vi "EvaluateLowRate.vi"(7 "Qbus":refnum<class "Qbus.lvclass">, 8 "error in (no error)":errorcluster, 9 "data":T1, 10 "new block number":u32, 11 "config":variant) -> (0 "error out":errorcluster, 1 "new data":T1, 2 "fire low rate data flow":bool, 3 "config out":variant)   [LabVIEW 2017, in "DataAccumulator.lvlib"]
uses:
  <vilib>/addons/InsightCM/Devices/Shared/Common/DataAccumulator/DataAccumulator.lvlib
  <vilib>/addons/InsightCM/Devices/Shared/Common/DataFlow/controls/Data.ctl
  <vilib>/addons/InsightCM/Utilities/DataAccessors/controls/wfmSGL_DVR.ctl
  <vilib>/addons/PointValueMap/controls/PointMap.ctl
  <vilib>/addons/InsightCM/Devices/Shared/Common/DataFlow/controls/Type.ctl
  <vilib>/addons/Qbus/Qbus.lvclass
  <vilib>/addons/InsightCM/Devices/Shared/Common/DataAccumulator/controls/DataStoreOps.ctl
  <vilib>/addons/InsightCM/Devices/Shared/Common/DVRBuffer/controls/BufferLocation.ctl
  <vilib>/addons/InsightCM/Devices/Shared/Common/DataAccumulator/controls/DataStoreType.ctl
  <vilib>/addons/InsightCM/Utilities/Analysis/Shared/controls/PulsePositions.ctl
  <vilib>/addons/InsightCM/Devices/Shared/Common/DataAccumulator/controls/BlockParams.ctl
  <vilib>/addons/InsightCM/Devices/Shared/Common/DVRBuffer/DVRBuffer.lvlib
  <vilib>/addons/PointValueMap/PointValueMap.lvlib
  <vilib>/addons/InsightCM/Devices/Shared/Common/DataFlow/DataFlow.lvlib
  <vilib>/addons/InsightCM/Utilities/Analysis/Shared/AnalysisHelper.lvlib
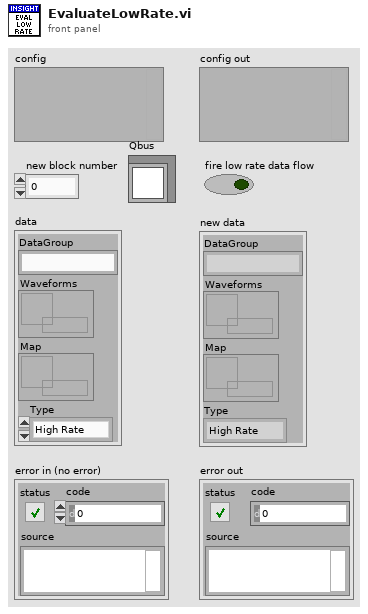
[diagram p1: front panel]
types:
  T1 = typedef "DataFlow.lvlib/Data.ctl" = cluster{"DataGroup":string, "Waveforms":T2, "Map":T3, "Type":T4}
  T2 = typedef "wfmSGL_DVR.ctl" = refnum<data-value>
  T3 = typedef "PointValueMap.lvlib/PointMap.ctl" = refnum<data-value>
  T4 = typedef "DataFlow.lvlib/Type.ctl" = enum16{"High Rate", "Low Rate", "Burst Mode"}
  T5 = typedef "DataAccumulator.lvlib/AccumulationSettings.ctl" = cluster{"Type":T6, "Length":dbl, "Max Time (sec)":dbl, "Start Block":T7, "Acquired (sec)":dbl, "Acquired (pulses)":i32, "Initial Pulse Offset":dbl, "Stop Block":T7, "LastBlockAdded":u32}
  T6 = typedef "DataAccumulator.lvlib/accumulationType.ctl" = enum16{"none", "seconds", "revolutions"}
  T7 = typedef "DVRBuffer.lvlib/BufferLocation.ctl" = cluster{"Block":u32, "Index":i32}
  T8 = typedef "DataAccumulator.lvlib/DataStoreOps.ctl" = enum16{"Reset", "Init", "Clear", "SetWfms", "GetWfms"}
  T9 = typedef "DataAccumulator.lvlib/DataStoreType.ctl" = cluster{"Group":string, "waveforms":waveform(sgl)[], "pulse positions array":T10[], "start block":T7}
  T10 = typedef "AnalysisHelper.lvlib/PulsePositions.ctl" = cluster{"Name":string, "Pulse Position Data":dbl[], "Pulses Per Rev":i32}
  T11 = typedef "DataAccumulator.lvlib/BlockParams.ctl" = cluster{"start block":T7, "stop block":T7, "BlockSizeSeconds":dbl}
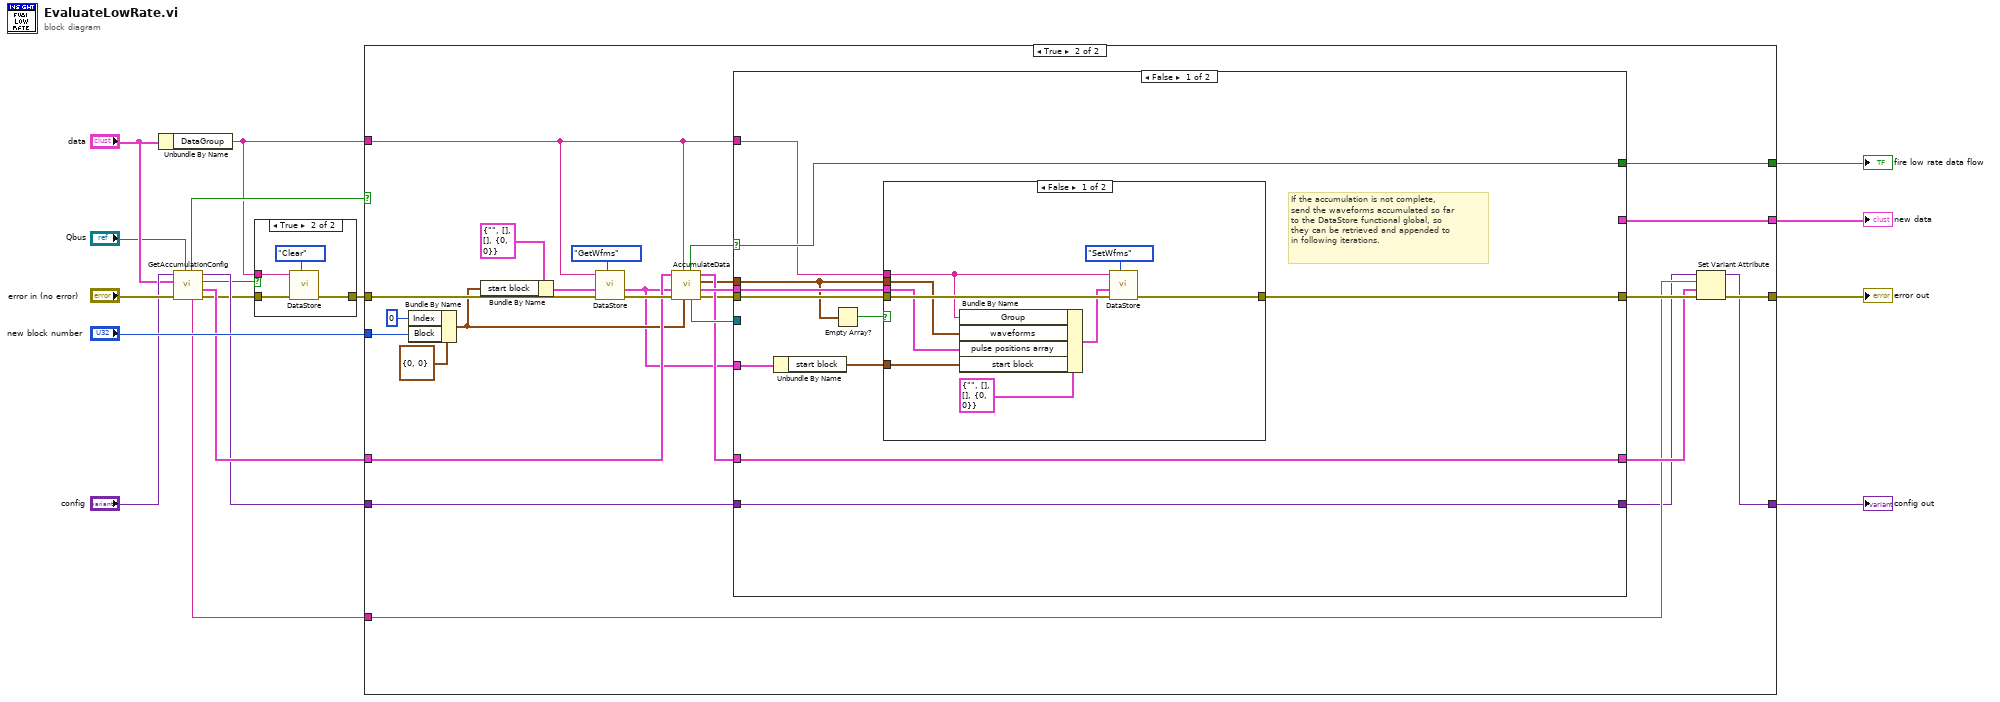
[diagram p0: block diagram]
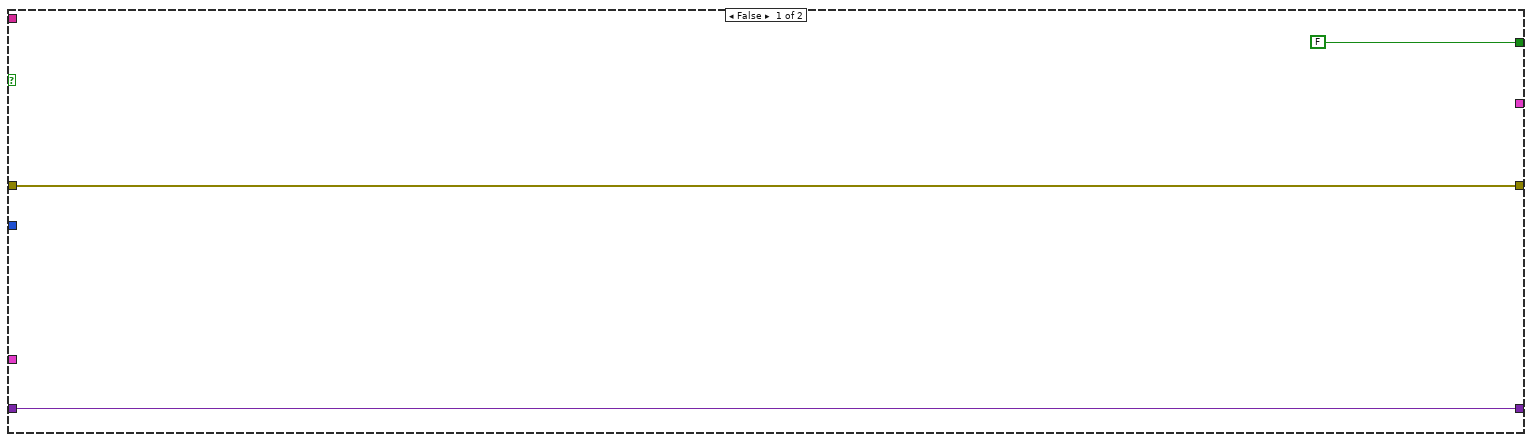
[diagram p2: hidden frame]
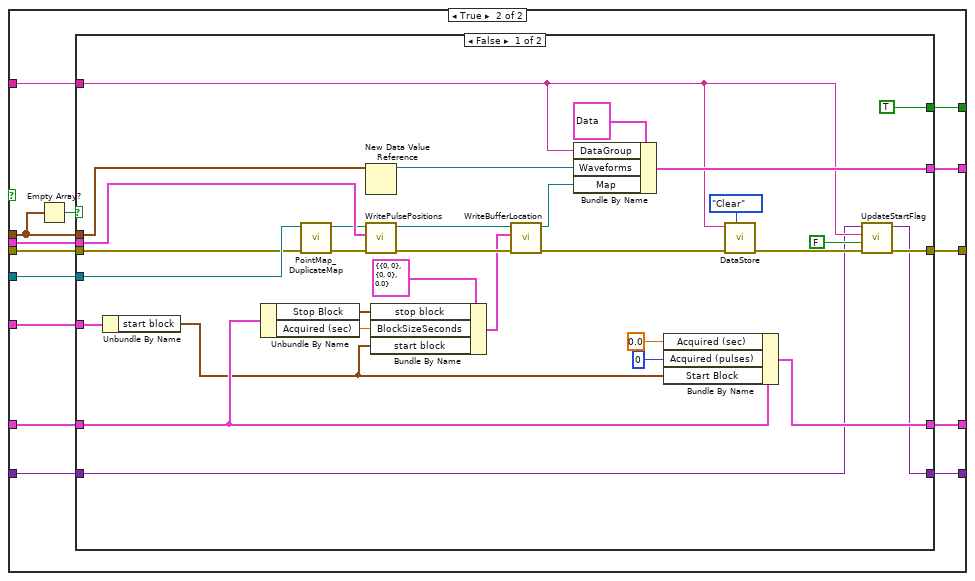
[diagram p4: hidden frame]
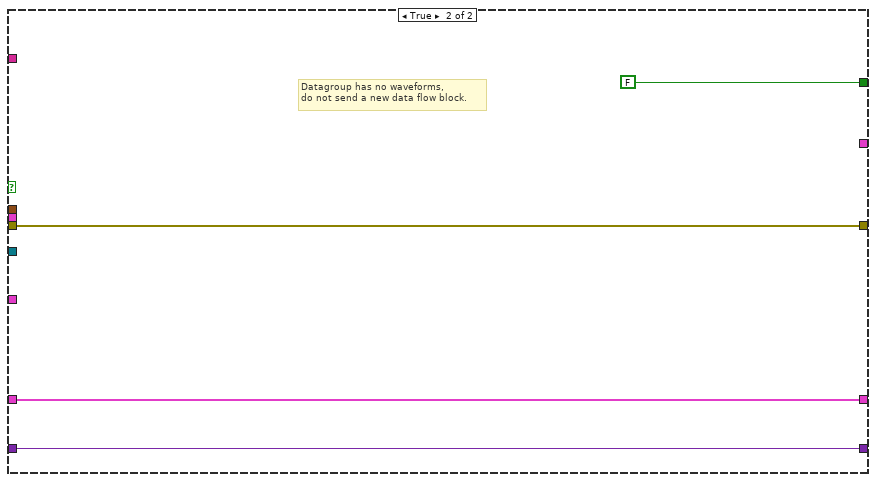
[diagram p5: hidden frame]
diagram:
  n1 = Unbundle By Name("data") -> ("DataGroup"=w4:string)
  n2 = call <vilib>:"GetAccumulationConfig.vi"("Qbus"="Qbus", "error in (no error)"="error in (no error)", "data"="data", "config"="config") -> ("error out"=w3:errorcluster, "accumulation settings"=w10:T5, "clear buffer"=w1:bool, "config"=w8:variant, "accumulation settings key"=w6:string, "ok to start"=w9:bool)  [unwired: 2 in]
  n3 = case shown="True" w1 {
    tunnel: w3 -> [w18 w21]
    tunnel: [w18 w20] -> w2
    tunnel: w4 -> [_ w19]
    frame False {
    }
    frame True {
      n4 = call <vilib>:"DataStore.vi"("operation"=DataStoreOps."Clear", "error in (no error)"=w21, "group"=w19) -> ("error out"=w20:errorcluster)  [unwired: 7 in, 1 out]
    }
  }
  n5 = case shown="True" w9 {
    tunnel: "new block number" -> [_ w27]
    tunnel: w2 -> [w25 w32]
    tunnel: w8 -> [w24 w34]
    tunnel: [_ w49] -> w15
    tunnel: [FALSE w47] -> w14
    tunnel: w4 -> [_ w35]
    tunnel: [w25 w42] -> w13
    tunnel: [w24 w41] -> w12
    tunnel: w10 -> [_ w37]
    tunnel: w6 -> [_ w36]
    frame False {
    }
    frame True {
      n6 = Bundle By Name(cluster=T7 {"Block"=0, "Index"=0} ("new block"), "Index"=0, "Block"=w27) -> (w29:T7)
      n7 = Bundle By Name(cluster=T9 {"Group"="", "waveforms"=[], "pulse positions array"=[], "start block"={"Block"=0, "Index"=0}} ("data in"), "start block"=w29) -> (w30:T9)
      n8 = call <vilib>:"DataStore.vi"("operation"=DataStoreOps."GetWfms", "error in (no error)"=w32, "data in"=w30, "group"=w35) -> ("error out"=w39:errorcluster, "data out"=w28:T9)  [unwired: 6 in]
      n9 = call <vilib>:"AccumulateData.vi"("new block"=w29, "data group"=w35, "error in (no error)"=w39, "data in"=w28, "accumulation settings"=w37) -> ("error out"=w44:errorcluster, "pulse positions array"=w50:T10[], "waveforms"=w45:waveform(sgl)[], "accumulation settings out"=w46:T5, "most recent map"=w51:T3, "accumulation complete"=w48:bool)  [unwired: 1 in]
      n10 = case shown="False" w48 {
        selector: w48 -> [w63 _]
        tunnel: w51 -> [_ w87]
        tunnel: w44 -> [w61 w81]
        tunnel: [w60 w86] -> w43
        tunnel: w50 -> [w62 w85]
        tunnel: [_ w84] -> w49
        tunnel: [w63 w80] -> w47
        tunnel: w35 -> [w58 w82]
        tunnel: w45 -> [w55 w78]
        tunnel: w46 -> [w59 w83]
        tunnel: [w59 w77] -> w40
        tunnel: w34 -> [w57 w76]
        tunnel: [w57 w75] -> w33
        tunnel: w28 -> [w54 w74]
        frame False {
          # "If the accumulation is not complete,\nsend the waveforms accumulated so far\nto the DataStore functional global, so\nthey can be retrieved and appended to\nin following iterations."
          n11 = Unbundle By Name(w54) -> ("start block"=w53:T7)
          n12 = Empty Array?(array=w55) -> (empty?=w56:bool)
          n13 = case shown="False" w56 {
            tunnel: w55 -> [w67 _]
            tunnel: w62 -> [w68 _]
            tunnel: w61 -> [w72 w73]
            tunnel: [w71 w73] -> w60
            tunnel: w58 -> [w64 _]
            tunnel: w53 -> [w65 _]
            frame False {
              n14 = Bundle By Name(cluster=T9 {"Group"="", "waveforms"=[], "pulse positions array"=[], "start block"={"Block"=0, "Index"=0}} ("data in"), "Group"=w64, "waveforms"=w67, "pulse positions array"=w68, "start block"=w65) -> (w66:T9)
              n15 = call <vilib>:"DataStore.vi"("operation"=DataStoreOps."SetWfms", "error in (no error)"=w72, "data in"=w66, "group"=w64) -> ("error out"=w71:errorcluster)  [unwired: 6 in, 1 out]
            }
            frame True {
            }
          }
        }
        frame True {
          n16 = Empty Array?(array=w78) -> (empty?=w79:bool)
          n17 = case shown="False" w79 {
            tunnel: w87 -> [w118 _]
            tunnel: [w95 w119] -> w86
            tunnel: w85 -> [w112 _]
            tunnel: [w117 _] -> w84
            tunnel: w78 -> [w113 _]
            tunnel: w81 -> [w90 w119]
            tunnel: w83 -> [w109 w121]
            tunnel: w82 -> [w93 _]
            tunnel: [TRUE FALSE] -> w80
            tunnel: [w114 w121] -> w77
            tunnel: w76 -> [w92 w120]
            tunnel: [w91 w120] -> w75
            tunnel: w74 -> [w89 _]
            frame False {
              n18 = Unbundle By Name(w89) -> ("start block"=w88:T7)
              n19 = Unbundle By Name(w109) -> ("Stop Block"=w99:T7, "Acquired (sec)"=w100:dbl)
              n20 = call <vilib>:"PointMap_DuplicateMap.vi"("error in (no error)"=w90, "map in"=w118) -> ("error out"=w104:errorcluster, "duplicate map"=w105:T3)  [unwired: 8 in]
              n21 = New Data Value Reference(data value=w113) -> (data value reference=w102:refnum<data-value>)  [unwired: 1 in, 1 out]
              n22 = call <vilib>:"WritePulsePositions.vi"("error in (no error)"=w104, "pulse positions array"=w112, "map in"=w105) -> ("error out"=w107:errorcluster, "map out"=w106:T3)  [unwired: 7 in]
              n23 = Bundle By Name(cluster=T11 {"start block"={"Block"=0, "Index"=0}, "stop block"={"Block"=0, "Index"=0}, "BlockSizeSeconds"=0.0} ("BlockParams"), "stop block"=w99, "BlockSizeSeconds"=w100, "start block"=w88) -> (w98:T11)
              n24 = call <vilib>:"WriteBufferLocation.vi"("error in (no error)"=w107, "block params"=w98, "map in"=w106) -> ("error out"=w111:errorcluster, "map out"=w101:T3)  [unwired: 7 in]
              n25 = Bundle By Name(cluster=T1 {"DataGroup"="", "Waveforms"=refnum, "Map"=refnum, "Type"=enum."High Rate"} ("data"), "DataGroup"=w93, "Waveforms"=w102, "Map"=w101) -> (w117:T1)
              n26 = Bundle By Name(cluster=w109, "Acquired (sec)"=0.0, "Acquired (pulses)"=0, "Start Block"=w88) -> (w114:T5)
              n27 = call <vilib>:"DataStore.vi"("operation"=DataStoreOps."Clear", "error in (no error)"=w111, "group"=w93) -> ("error out"=w96:errorcluster)  [unwired: 7 in, 1 out]
              n28 = call <vilib>:"UpdateStartFlag.vi"("error in (no error)"=w96, "BlkComplete"=FALSE, "group"=w93, "config"=w92) -> ("error out"=w95:errorcluster, "config"=w91:variant)  [unwired: 6 in]
            }
            frame True {
              # "Datagroup has no waveforms,\ndo not send a new data flow block."
            }
          }
        }
      }
      n29 = Set Variant Attribute(Variant=w33, name=w36, value=w40, error in=w43) -> (Variant out=w41:variant, error out=w42:errorcluster)  [unwired: 1 out]
    }
  }
  "fire low rate data flow" <- w14
  "new data" <- w15
  "error out" <- w13
  "config out" <- w12
